vi "Configure Trigger Model Delta Branch.vi"(6 "Measurement Block":i32=1 min=1 format="%#.6g", 7 "Branch To Block":i32=1 min=1 format="%#.6g", 8 "error in (no error)":errorcluster, 9 "Target Difference":dbl=1.0 min=1.0 format="%#.6g", 10 "Block Number (1)":i32=1 min=1 format="%#.6g", 11 "VISA resource name":refnum<visa-resource-name>) -> (0 "error out":errorcluster, 3 "VISA resource name out":refnum<visa-resource-name>)   [LabVIEW 2021, in "Keithley DMM7510.lvlib"]
doc: "This VI defines a trigger model block that goes to a specified block if the difference of two measurements meets preset criteria."
uses:
  Keithley DMM7510.lvlib
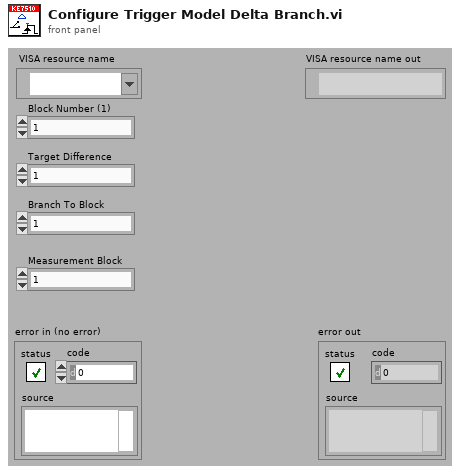
[diagram p1: front panel]
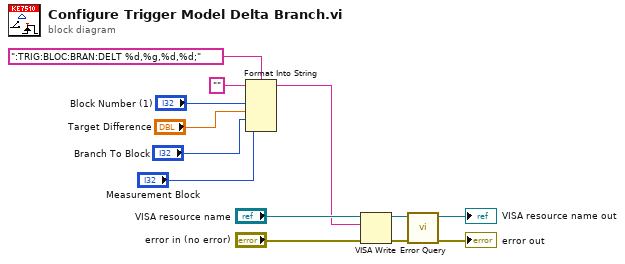
[diagram p0: block diagram]
diagram:
  n1 = Format Into String(format string=":TRIG:BLOC:BRAN:DELT %d,%g,%d,%d;", initial string="", "Block Number (1)", "Target Difference", "Branch To Block", "Measurement Block") -> (resulting string=w4:string)  [unwired: 1 in, 1 out]
  n2 = VISA Write(VISA resource name="VISA resource name", write buffer=w4, error in (no error)="error in (no error)") -> (VISA resource name out=w9:refnum<visa-resource-name>, error out=w8:errorcluster)  [unwired: 1 out]
  n3 = call "Error Query.vi"("error in (no error)"=w8, "VISA resource name"=w9) -> ("error out"=→"error out":errorcluster, "VISA resource name out"=→"VISA resource name out":refnum<visa-resource-name>)  [unwired: 8 out]
